vi "Add String to HashTable.vi"(8 "error in (no error)":errorcluster caption="错误输入（无错误）", 9 "Value":string, 10 "Name":string, 11 "Contstant Base 输入":refnum<class "Tag Data.lvclass"> caption="DNL_LabVIEW Object in") -> (0 "error out":errorcluster caption="错误输出", 3 "Contstant Base 输出":refnum<class "Tag Data.lvclass"> caption="DNL_LabVIEW Object out")   [LabVIEW 2013, in "Tag Data.lvclass"]
uses:
  Tag Data.lvclass
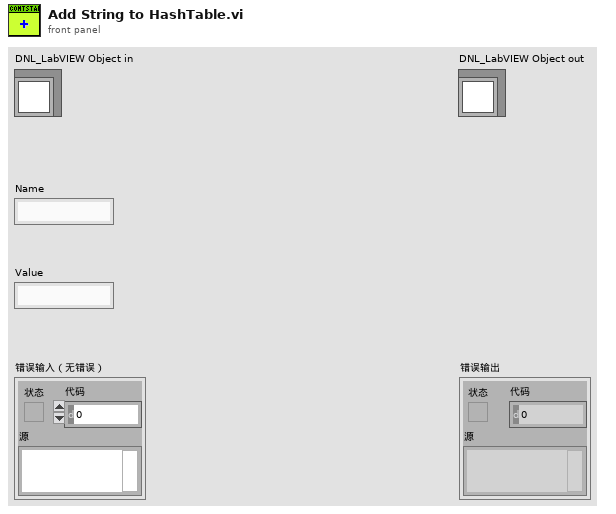
[diagram p1: front panel]
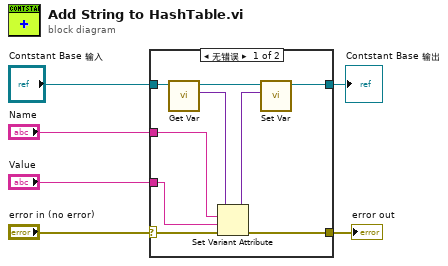
[diagram p0: block diagram]
diagram:
  n1 = case shown="无错误" "error in (no error)" {
    selector: "error in (no error)" -> [w10 w17]
    tunnel: [w9 w17] -> w5
    tunnel: [w11 w16] -> w3
    tunnel: "Contstant Base 输入" -> [w15 w16]
    tunnel: "Name" -> [w8 _]
    tunnel: "Value" -> [w7 _]
    frame No Error {
      n2 = call-dynamic "Get Var.vi"("Contstant Base输入"=w15) -> ("Var"=w14:variant, "Contstant Base输出"=w12:refnum<class "Tag Data.lvclass">)  [unwired: 8 in, 1 out]
      n3 = Set Variant Attribute(Variant=w14, name=w8, value=w7, error in=w10) -> (Variant out=w13:variant, error out=w9:errorcluster)  [unwired: 1 out]
      n4 = call-dynamic "Set Var.vi"("Var"=w13, "Contstant Base输入"=w12) -> ("Contstant Base输出"=w11:refnum<class "Tag Data.lvclass">)  [unwired: 8 in, 1 out]
    }
    frame Error {
    }
  }
  "error out" <- w5
  "Contstant Base 输出" <- w3
